vi "nnfft.vi"() -> ()   [LabVIEW 2014]
uses:
  <vilib>/imath/engines/lvmath/Functions/Error Handling/error.ctl
  <vilib>/Analysis/baseanly.llb/Real A x B.vi
  <vilib>/DAQmx/create/channels.llb/DAQmx Create Channel (AI-Voltage-Basic).vi
  <vilib>/DAQmx/create/channels.llb/DAQmx Create Channel (DO-Digital Output).vi
  <vilib>/imath/engines/lvmath2/RunTimeEngine/Managers/WorkSpace/UID Generator.vi
  <vilib>/imath/engines/lvmath2/RunTimeEngine/NonStaticBuiltInFunctions/Manual/NIMS_NS_load.vi
  <vilib>/imath/engines/lvmath/Plug In/Control Design/NonStaticBuiltInFunctions/NIMS_NS_length.vi
  <vilib>/imath/engines/lvmath/Plug In/_Char/NIMS_CH_String to Character Array.vi
  <vilib>/imath/engines/lvmath2/RunTimeEngine/RunTimeType/NIMS_RunTimeType_From StrictType (excl LVString).vi
  <instcachedir>/0/NIMS_RunTimeType_From StrictType (excl LVString)_15A5391EEA9C4AACB9955AC755B83D29.lvgen/NIMS_RunTimeType_From StrictType (excl LVString)_15A5391EEA9C4AACB9955AC755B83D29_001.vi
  <vilib>/imath/engines/lvmath2/RunTimeEngine/Managers/SymbolTable/Write Variable.vi
  <vilib>/imath/engines/lvmath2/RunTimeEngine/RunTimeSymbolToken/NIMS_RunTimeSymbolToken_ReadVariable-1out.vi
  <vilib>/imath/engines/lvmath/Plug In/Control Design/RunTimeSymbolToken/NIMS_CD_RunTimeSymbolToken_ResolveSymbol.vi
  <instcachedir>/0/NIMS_CD_RunTimeSymbolToken_ResolveSymbol_41E3A8865B50468190B6702AA519A4CE.lvgen/NIMS_CD_RunTimeSymbolToken_ResolveSymbol_41E3A8865B50468190B6702AA519A4CE_000.vi
  <instcachedir>/0/NIMS_CD_RunTimeSymbolToken_ResolveSymbol_41E3A8865B50468190B6702AA519A4CE.lvgen/NIMS_CD_RunTimeSymbolToken_ResolveSymbol_41E3A8865B50468190B6702AA519A4CE_001.vi
  <vilib>/imath/engines/lvmath/Plug In/Control Design/RunTimeSymbolToken/NIMS_CD_RunTimeSymbolToken_ResolveUDForVariable-1out.vi
  <vilib>/imath/engines/lvmath/Plug In/Control Design/ArithmeticOperatorToken/NIMS_CD_NS_ArithmeticOperator_minus.vi
  <vilib>/imath/engines/lvmath/Plug In/Control Design/ArithmeticOperatorToken/NIMS_CD_NS_ArithmeticOperator_cctranspose.vi
  <vilib>/imath/engines/lvmath2/RunTimeEngine/CommandStatement/NIMS_CommandStatement_MaskErr.vi
  <vilib>/imath/engines/lvmath2/RunTimeEngine/Managers/SymbolTable/Read Variable.vi
  <vilib>/imath/engines/lvmath2/RunTimeEngine/RunTimeType/NIMS_RunTimeType_Get Case Value.vi
  <vilib>/imathl/engines/lvmath/Functions/Error Handling/Create Error.vi
  <vilib>/imath/engines/lvmath2/RunTimeEngine/RunTimeType/NIMS_RunTimeType_To Numeric.vi
  <instcachedir>/0/NIMS_RunTimeType_To Numeric_CEDD3DBADEB64FB59CD8C53099B6B149.lvgen/NIMS_RunTimeType_To Numeric_CEDD3DBADEB64FB59CD8C53099B6B149_000.vi
  <vilib>/imath/engines/lvmath2/RunTimeEngine/NodeEndStatement/NIMS_NodeEndStatement_Get Scalar.vi
  <instcachedir>/0/NIMS_NodeEndStatement_Get Scalar_62223508BC7F4CFFA0F66459A43A6646.lvgen/NIMS_NodeEndStatement_Get Scalar_62223508BC7F4CFFA0F66459A43A6646_000.vi
  <vilib>/imath/engines/lvmath/Plug In/_Char/RunTimeType/NIMS_CH_RunTimeType_To Character 2D.vi
  <instcachedir>/0/NIMS_NodeEndStatement_Get Scalar_62223508BC7F4CFFA0F66459A43A6646.lvgen/NIMS_NodeEndStatement_Get Scalar_62223508BC7F4CFFA0F66459A43A6646_001.vi
  <vilib>/Analysis/Matrix/Numeric/Conversions/Array To Matrix - RA2.vi
  <vilib>/imath/engines/lvmath/Plug In/_Char/NIMS_CH_Character 2D to U8 2D.vi
  <vilib>/imath/engines/lvmath/Functions/Error Handling/MergeErrorsWrapper.vi
  <vilib>/imath/engines/lvmath2/RunTimeEngine/NodeEndStatement/MC_NodeEndStatement_Dispose.vi
  <vilib>/imath/engines/lvmath2/RunTimeEngine/NodeEndStatement/NIMS_NodeEndStatement_Output.vi
  <instcachedir>/0/NIMS_NodeEndStatement_Output_53EC0D466D134D7ABD903AC30B43404B.lvgen/NIMS_NodeEndStatement_Output_53EC0D466D134D7ABD903AC30B43404B_013.vi
  <instcachedir>/0/NIMS_NodeEndStatement_Output_53EC0D466D134D7ABD903AC30B43404B.lvgen/NIMS_NodeEndStatement_Output_53EC0D466D134D7ABD903AC30B43404B_011.vi
  <instcachedir>/0/NIMS_NodeEndStatement_Output_53EC0D466D134D7ABD903AC30B43404B.lvgen/NIMS_NodeEndStatement_Output_53EC0D466D134D7ABD903AC30B43404B_001.vi
  <instcachedir>/0/NIMS_NodeEndStatement_Output_53EC0D466D134D7ABD903AC30B43404B.lvgen/NIMS_NodeEndStatement_Output_53EC0D466D134D7ABD903AC30B43404B_012.vi
  <vilib>/imath/engines/lvmath2/RunTimeEngine/ErrorHandling/NIMS_Finalize Error.vi
  <vilib>/DAQmx/configure/timing.llb/DAQmx Timing (Sample Clock).vi
  <vilib>/DAQmx/read.llb/DAQmx Read (Analog 1D Wfm NChan NSamp).vi
  <vilib>/express/express analysis/Spectral/Block/exnSpectralBlock spectral measurements PSD poly.vi
  <vilib>/express/express analysis/Spectral/Block/exnSpectralBlock spectral measurements PSD WFM.vi
  <vilib>/Analysis/Matrix/Numeric/Conversions/Array To Matrix - RA.vi
  <vilib>/Analysis/Matrix/Numeric/Add/Add - RM,RM.vi
  <vilib>/DAQmx/write.llb/DAQmx Write (Digital 2D Bool NChan 1Samp NLine).vi
  <vilib>/express/express analysis/Spectral/XNode/ExpressSpectralMeasurementsBlockNode.xnode
  <vilib>/Analysis/Matrix/NI_Matrix.lvlib
  <vilib>/Analysis/NI_AALBase.lvlib
  <vilib>/imath/engines/lvmath2/RunTimeEngine/Managers/SymbolTable/NIMS_WorkSpace.lvlib
panel:
  out "detected signal":i16[][](graph)
  out "Max power":dbl
  out "Waveform Chart":waveform(dbl)[](graph)
  out "canonical signal":i16(graph)
  in  "Path":path=path "Z:/v/birds/align/net_detector_0.28_0.775.mat"
  in  "stop":bool
  out "FFT_TIME_SHIFT":dbl=0.005
  out "FFT_SIZE":i32=256
  out "samplerate":dbl=24414.0625
  out "window":dbl[][](graph)=[[-72.97635032393673, -73.52535220045053, -65.72887335245875, -68.76871345390529, -72.8382109706844, -72.4284168123761, -76.29548482618758, -74.74287956205296, -81.97895834534424, -76.96305090475649, -75.98014073911352, -80.03992621585844, -83.84107312947093, -89.59209404799233, -79.87440020414152, -81.36512283954667, -88.18744053916166, -81.6924166622812, -77.53707705274705, -86.56451602394448, -79.73285708058553, -74.22115387848037, -71.41210134154478, -74.47517384018045, -74.77033095311324, -80.80005153541933, -80.79191388333305, -77.97946550843649, -75.05698688298563, -77.91422524584947, -81.26748634507513, -78.23409719434568, -71.56701464425281, -69.17263385066326, -77.53908052412173, -75.51920407149245, -72.81493380643417, -75.82836580399663, -79.16788759874976, -85.18140498406765, -73.69950641565677, -77.89257807943649, -89.09322579355587, -86.98629885093659, -82.38468041348978, -80.6411265118298, -82.76696738280094, -88.62107664481837, -80.16920149619398, -87.78502444899082, -76.5547272830016, -79.26058810386263, -83.94947298172212], [-66.67637324595356, -64.45280082019433, -72.37911061109125, -80.94357987532189, -72.53604430129853, -77.45470711834774, -89.59806575492826, -76.48927163271915, -73.61448223145683, -73.49144401291508, -71.27370666896533, -71.20261780246133, -74.92587625827385, -74.29334726263828, -76.65530048928724, -82.00140588849537, -79.57538322888249, -77.80520492576613, -81.78737082190267, -81.793811852895, -76.25688370577186, -78.13061054962415, -79.77815579754174, -74.3873327071945, -75.70646544653732, -90.72121289782154, -78.03321007215462, -81.03438405652348, -79.87658452660123, -76.00205540897467, -89.87308398872139, -81.86767670866956, -76.2852996579092, -70.93465158513496, -71.34523644690213, -79.93221348833194, -92.79662932893322, -79.70914845480407, -80.2829643889263, -84.90892181441768, -76.68651665541584, -84.51267326878296, -82.8204756496925, -76.73565845150263, -73.04092896348672, -74.3315440085461, -78.03729006688118, -81.70866916339699, -92.11943263220843, -79.10810077302251, -80.08002292830199, -86.99321689797517, -85.04323742707173], [-60.36185307894806, -67.68102358288463, -73.44778253010914, -83.24181048562586, -73.96144044519264, -84.69635305857125, -81.14261573322445, -79.25621064770326, -76.529695092035, -75.04627154406595, -73.90530564973237, -75.82555328376658, -72.10380949692679, -75.32839456413583, -76.50304991511011, -75.65339129055367, -77.00187973819256, -76.57898166561162, -82.8025996290185, -73.19174517705048, -69.09785163927901, -67.53276211170689, -72.94360264826646, -79.97186045768333, -88.56886550153519, -88.83521591582405, -76.65307428710892, -73.00745577396138, -74.258180742689, -71.06328438122829, -72.78097301088393, -76.66465643284776, -81.62018899033966, -75.65821895156606, -82.17348753133518, -80.91069867191484, -70.46021775773852, -68.83368607770463, -69.03429126209139, -72.72415945910303, -73.80156036987256, -69.28349217732242, -68.01356058946793, -73.4812440368461, -75.17978018102508, -77.01602519651868, -73.18724221539284, -73.00676255493443, -71.9944333961078, -72.09084959215544, -78.65722374826107, -76.66612517006482, -74.38697175839361], [-86.00798842509802, -75.66491243286761, -69.45998734378524, -75.90898538704424, -71.26588425831507, -68.18490140120666, -76.40500842112715, -90.04695090636658, -75.34084116331435, -73.50738067142525, -78.60366511108383, -81.21647416858836, -78.9684969474276, -82.40208977563746, -73.24305990075133, -71.12237211198403, -82.91234590794866, -80.93715499149765, -78.06474769268046, -75.91020347678767, -81.60811248967987, -82.86113678420863, -76.87398598776707, -74.38664233198445, -71.82140107556668, -74.67033624127943, -78.17390364475995, -72.60207540814541, -71.04336646832618, -67.87557323613137, -67.16318617639155, -69.4250953016462, -71.39893400102616, -68.4807322912351, -82.25308112419869, -68.3200120825788, -69.81250624283365, -71.84163203711881, -66.75402172042715, -86.50070599392079, -68.88587550717388, -64.27484144399455, -63.21158787522782, -66.63527192363303, -67.84532057406827, -66.45376461718031, -67.62579522979001, -70.50214513926198, -67.25446907463098, -65.19333416310778, -69.41880953289862, -71.51704770295385, -69.35219267630163], [-84.02423956482974, -80.30370937609739, -72.07006291884605, -78.91836472420934, -68.25364204650245, -76.68501322644221, -75.18375824555125, -71.83467956160965, -70.95375248124259, -74.08077326369566, -67.38027814308849, -72.93566891736185, -67.65115715678446, -64.85035252961103, -64.82034005578986, -70.26034479840374, -70.45877563236849, -76.54420720294256, -81.78534267236304, -78.15256514501289, -82.91835245277196, -72.46741612058328, -73.68274550784452, -78.34739661909776, -78.9666065362011, -77.78534451234053, -74.37093982228039, -74.12317719447532, -78.16971177499396, -74.52074730296583, -76.54045500868807, -75.84578212694746, -74.67082902652055, -77.18938861537275, -69.907454938437, -75.34017205802814, -79.50572953621057, -72.34299872242158, -78.18111149918124, -75.54782414585868, -80.561212592933, -75.11175049302021, -75.69417919582135, -78.60245860449001, -95.87767775375552, -87.11569980194378, -85.92469188794526, -77.60906632245548, -71.79465409556695, -77.42305609850067, -83.12532465877507, -77.05370659978007, -79.71270482455323], [-81.65381289229904, -83.21306508163494, -79.67200080348587, -70.22488500380918, -67.822116429376, -66.63216387482694, -69.55869616362561, -81.4902489378859, -78.79527713122093, -67.33672711847055, -60.3507452058667, -58.73683599716651, -60.551256165403004, -64.32429540525435, -64.72915177181335, -66.22450762492544, -91.58683040813399, -84.38309032351134, -73.15703222555902, -67.56828517210809, -73.57402369414261, -74.61227498203642, -77.96234972672107, -71.20169596754377, -67.59425187404017, -71.05072968837761, -76.59202882173123, -80.82688050565231, -73.80977565569785, -74.11008150826325, -71.41495591144026, -77.7753259840453, -76.2037224219869, -79.29218960734961, -91.32887569169418, -85.7301249007533, -80.85079471385804, -74.18909859098636, -72.26476740645808, -73.32812816132918, -75.76304038496815, -77.50309269541718, -73.05090728588225, -71.86574972197677, -70.43058663023983, -70.27591438296898, -74.08700994335328, -73.95177555941575, -91.88200670928885, -81.81331742651899, -78.5318263177664, -71.72863325861373, -74.46402142105174], [-68.9073260193967, -67.48746628924823, -77.17977545292486, -73.64769729099787, -72.22314785727713, -70.87731592806281, -70.716894114705, -81.05789728768389, -71.43183739761903, -73.18594956271083, -69.20692855319716, -68.67815172293385, -53.670962574687195, -50.933292802391094, -61.63077047269332, -71.38477936140977, -99.14569301468815, -72.06562278900773, -74.1511754276874, -76.89887661322872, -72.58638083106267, -75.05922049222346, -77.77343214730914, -75.92379207288955, -71.20325396519463, -76.43168692677789, -82.39119805432924, -71.51193816622407, -73.1364143798586, -78.71213040493862, -94.96695151435625, -74.49648076734441, -69.43231860114312, -70.3883036388338, -76.6904252867458, -85.10664073795765, -83.20367116345437, -79.50305757838471, -74.03353087441471, -78.99092469951292, -91.58509571109497, -91.89444165362694, -79.83050377520397, -79.27431251753544, -84.8477925073274, -72.43027174269308, -65.52053141156405, -66.12640598342038, -76.108195822798, -89.27574855580932, -70.90463844447619, -66.46347719708304, -72.98967833873088], [-73.0439648592936, -70.44453567604373, -79.75314488295, -80.07642120248778, -78.37070295298031, -73.1201693139319, -78.53710949103558, -79.79936428129609, -79.86525021136373, -72.22971430283177, -67.84318418359742, -72.87558430802864, -53.003002816738515, -47.84968331998619, -50.98562535099076, -58.11218860294475, -61.60082326832688, -68.69125001358182, -70.44497259313596, -69.84352221154673, -72.07552086745858, -73.19525392036374, -85.84209460576159, -78.78668117995774, -108.96094371547589, -76.45977938927919, -75.02269494673682, -81.13939454241775, -76.23809744857965, -79.98125590046457, -85.47323069676317, -82.94387240494945, -77.0798993807903, -87.45325755760888, -74.60902178190632, -71.49002838584563, -72.65326888909527, -74.30285347007833, -71.51996549981243, -70.58127271813062, -67.50879993296408, -66.96776504010182, -67.5977737300707, -63.43592929677993, -65.07886006448592, -68.14664606850042, -65.25796945257115, -63.375993543512465, -69.69409051293428, -66.76473458025286, -67.28346558898642, -70.59116729035524, -67.66948910837607], [-68.77569667006642, -69.18302500016709, -71.01858086817602, -72.38028122261937, -69.84097809370121, -70.94893664271633, -76.08982385135212, -78.69559608023533, -75.44131958210247, -70.6072977643919, -68.94517408706297, -69.39438458347952, -63.31192689032822, -62.17555246766285, -67.17754626637941, -75.62442591074503, -78.75800065905979, -75.17375793297293, -73.35352004961631, -76.14826387288446, -76.94316620614036, -82.59526691265685, -71.38733095904792, -72.56519374181563, -83.3950501348429, -90.47654618015734, -84.51605264553925, -75.11223707596085, -75.67115447672266, -79.48878198359742, -72.8312370379487, -73.12224612826401, -73.48400779569472, -72.78689045619967, -76.92547768121204, -78.40592890718482, -73.2310717836559, -66.03581732569029, -72.47607194397511, -63.68851741665692, -64.64949331188906, -58.02441919784529, -59.84253402809921, -55.317855401116205, -55.64943410315087, -55.07048062012055, -53.75573935219861, -59.01222904078905, -56.55051323885307, -55.924357615058895, -55.62810503061498, -54.23211672544804, -55.50519500194375], [-74.75832710617124, -75.4308719211877, -74.46594285292588, -73.08174465947688, -75.65741389741267, -76.85655422277733, -76.17724583134641, -78.7866469753405, -79.98861317568219, -81.89112371724251, -82.63604725769618, -83.140254780378, -81.67601959545613, -89.00653003380093, -88.73873918927613, -76.51543291625471, -75.79644478079794, -80.51350580935683, -78.29033538027453, -77.6006603336961, -82.29627474182139, -78.33191904398069, -75.62832998601185, -86.33820054880604, -78.0946880670678, -74.84100282711086, -75.24721439405523, -78.59378634737459, -82.46985087316023, -79.76367779929939, -83.59485868627448, -74.82964327789745, -83.47070996793212, -80.84481800459685, -88.96399452691867, -76.9164788840067, -70.71773824416289, -68.11387991161286, -84.5841447765394, -66.7959107046369, -68.75178657989372, -64.77026879341615, -67.70334881108903, -53.99229230247266, -54.15690890913606, -51.07210226513892, -47.4469848829612, -48.016313760511224, -46.89883581264472, -47.32639944655021, -47.087219879398575, -49.520586995280375, -51.40004089705311], [-84.80810487129318, -80.63211281718762, -78.56043117891872, -76.27943201998615, -77.15760293197748, -81.64091579144285, -83.57045080108676, -78.63130196693999, -81.47341405888328, -78.60904777055399, -78.00888189113262, -85.12607813424106, -83.64938163698022, -80.79078185456909, -81.96965893927523, -77.43741043097695, -78.52875304218192, -79.13790302072155, -79.8115060848578, -89.09700475707078, -79.84774992179518, -81.4208933359674, -79.45746012306984, -82.24946297830411, -87.56044829973484, -90.28729530511617, -76.44434861584307, -78.78897610507829, -93.34714140321714, -79.6437809904397, -77.08007637946908, -82.61823969652897, -96.96492301906731, -86.91840996208597, -78.2484679644696, -84.06167675912474, -80.58283631847846, -82.60282000113612, -80.08784422911889, -80.3818141223883, -71.63670327697784, -71.70751698739937, -76.76453620599743, -71.61768539867478, -69.32504730623252, -68.28032804698583, -65.759956184971, -65.61488756706426, -65.70881887875339, -67.262085308336, -71.32336101600086, -73.79617107128622, -74.47767495897709], [-74.24876447880565, -79.51183675628256, -89.46410450431294, -82.92587289022006, -77.7457556235718, -79.30413919682815, -80.50830335354752, -81.3585175894736, -71.63315075617669, -71.50011424611691, -78.47849160378934, -80.30674914126804, -73.11186901485297, -76.026499122226, -78.67243959562191, -81.28052088875201, -77.39332987892728, -79.17775124486431, -74.63358089302206, -74.2219431039591, -75.72536721687463, -78.63557830761712, -78.03300701227882, -78.73460743340698, -80.50182310318193, -74.34525414950886, -78.93836541260941, -97.94071592484138, -91.61898811661828, -78.45177452289117, -79.02722537868969, -87.81919073287318, -97.64889457820716, -86.08948913346865, -94.83472004300674, -80.29958208150036, -79.94308117838753, -87.26408456051925, -87.86724547094477, -77.22219882470283, -79.10106862704167, -81.9160924832359, -75.92381304866126, -79.29802559293336, -78.63678572865807, -80.2339821401618, -80.74035656476087, -75.34996964522848, -74.87202873304834, -76.5943391889857, -73.41497745912935, -75.30585362948747, -82.47751215796093], [-74.39306178800754, -73.02600059267387, -73.07393952038746, -74.9812550588737, -76.80613423181211, -79.21537174139556, -82.24804461952566, -79.88497680349332, -77.73780357707737, -76.38987395680789, -81.1372862629103, -84.67801257122353, -75.29730335181587, -84.00023147835932, -73.3237703431372, -74.21062661277206, -80.51423062939938, -73.23425723998423, -72.49958681733966, -80.41967028089522, -88.8780775783741, -79.02412566482069, -90.7377774207196, -73.42552841442792, -74.68738171044559, -73.67460705564318, -76.06590490239931, -84.7613317932862, -79.70125370326343, -79.49333540467144, -89.63642567674898, -83.03621171058427, -83.33948920260524, -82.46001987798482, -81.95215264151247, -85.35054456568888, -86.49328712600567, -81.97249680506789, -87.5387622178776, -85.66227087431446, -84.18576775722295, -80.40800661446254, -75.53107385453657, -82.15686513878657, -88.67483064056772, -87.66221780558206, -86.84772744676606, -79.53573628729012, -82.7762696782156, -80.7915757346325, -80.70452295791704, -85.6983850384739, -81.72315222245822], [-81.93627780778903, -76.28366916681793, -80.29872988619105, -87.05275862910486, -84.63141287821459, -77.18015134120228, -72.98884655283919, -75.52679661054356, -80.1056525653624, -74.6697942063844, -80.48729503314061, -75.50337131233141, -78.31665631669648, -82.43718806714023, -73.95226171890097, -72.9292996254482, -71.71861568455955, -80.7946502972628, -78.65549947452148, -76.96606097973789, -76.06401494770057, -75.97723913018525, -99.24458365039294, -75.64074011120537, -78.62239631692377, -86.48850642086873, -89.87032184925617, -82.76174629794922, -80.10136504583882, -79.9961860071702, -81.50677446791065, -84.25440065532206, -92.56018408560594, -83.18151695684361, -80.59299994282482, -83.02918337502582, -78.40907071643018, -77.83883198956002, -89.31961651857968, -76.63471365127987, -75.67292636105336, -81.12402945042773, -90.28605099784328, -79.706246286267, -84.4032682475605, -81.20491587848613, -83.58829972237129, -92.4308955170453, -114.2328518473521, -78.71042595894347, -73.75405245226335, -74.69214248881669, -80.75531088405972]]
  out "Full spectrogram":dbl[][](graph)=[[-60.61401215305423, -57.03689977091529, -62.342730493983005, -72.51114353592169, -76.22824519389013, -78.52855635448381, -79.58628749191288, -67.73644127838553, -68.84105664914598, -74.67612003437475, -75.63706315714897, -76.74817498515577, -78.32477078138152, -73.09465183010549, -84.9742009024476, -82.47248060505194, -73.7376673139534, -68.19154425689516, -69.20475014657619, -88.95954172279392, -72.41169373066344, -81.93627780778903, -76.28366916681793, -80.29872988619105, -87.05275862910486, -84.63141287821459, -77.18015134120228, -72.98884655283919, -75.52679661054356, -80.1056525653624, -74.6697942063844, -80.48729503314061, -75.50337131233141, -78.31665631669648, -82.43718806714023, -73.95226171890097, -72.9292996254482, -71.71861568455955, -80.7946502972628, -78.65549947452148, -76.96606097973789, -76.06401494770057, -75.97723913018525, -99.24458365039294, -75.64074011120537, -78.62239631692377, -86.48850642086873, -89.87032184925617, -82.76174629794922, -80.10136504583882, -79.9961860071702, -81.50677446791065, -84.25440065532206, -92.56018408560594, -83.18151695684361, -80.59299994282482, -83.02918337502582, -78.40907071643018, -77.83883198956002, -89.31961651857968, -76.63471365127987, -75.67292636105336, -81.12402945042773, -90.28605099784328, -79.706246286267, -84.4032682475605, -81.20491587848613, -83.58829972237129, -92.4308955170453, -114.2328518473521, -78.71042595894347, -73.75405245226335, -74.69214248881669, -80.75531088405972, -82.82888754576534, -82.01868690982059, -81.78786972713498, -82.23423354778731, -78.28473979595428, -80.87670751550114, -83.51180745110783, -82.69187002570317, -88.82008519429516, -75.98520288801285, -77.99668488932495, -87.62318296403504, -99.6141881068977, -81.81521098057642, -84.17434860926062, -76.06411102913623, -74.1198176945056, -81.12819699144072, -80.91815093081088, -78.14119584663972, -85.49724935291657, -91.38248083630508, -84.18310225258782, -84.77684376955226, -85.16944043858439, -79.9875938684393, -79.27633537810411, -81.02037581981868, -81.35173013966018, -96.42412550048378, -90.54677478925467, -87.40674735535208, -88.1750427749852, -81.74631327698087, -82.23000371533317, -81.3297319022112, -76.40113644324768, -87.80400336917077, -78.37126070791032, -83.49976513431899, -80.51126278317908, -78.30520883073534, -76.75167662319735, -75.54421920890346, -79.45387512183294, -79.23147015013464, -82.63339787200022, -84.67740230235428, -67.26543692771294, -65.23077893430924, -76.87705017438371, -86.75690272003072, -85.56129846796406, -79.28978800654977]]
  out "in-loop read error":errorcluster
  out "daq create error":errorcluster
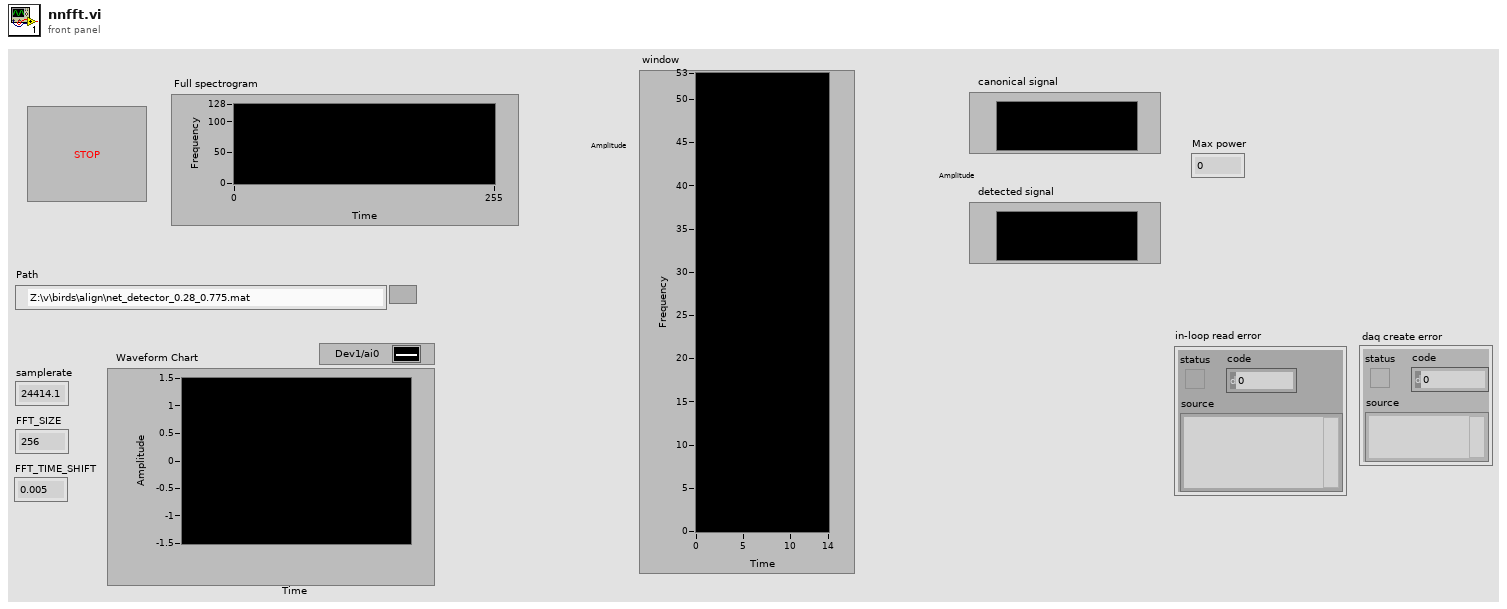
[diagram p1: front panel]
types:
  T1 = typedef "NI_Matrix.lvlib/RealMatrix.ctl" = dbl[][]
  T2 = cluster{"averaging mode":u16, "weighting mode":u16, "number of averages":u32}
  T3 = cluster{"dB On (F)":bool, "unwrap phase (F)":bool, "convert to degree (F)":bool}
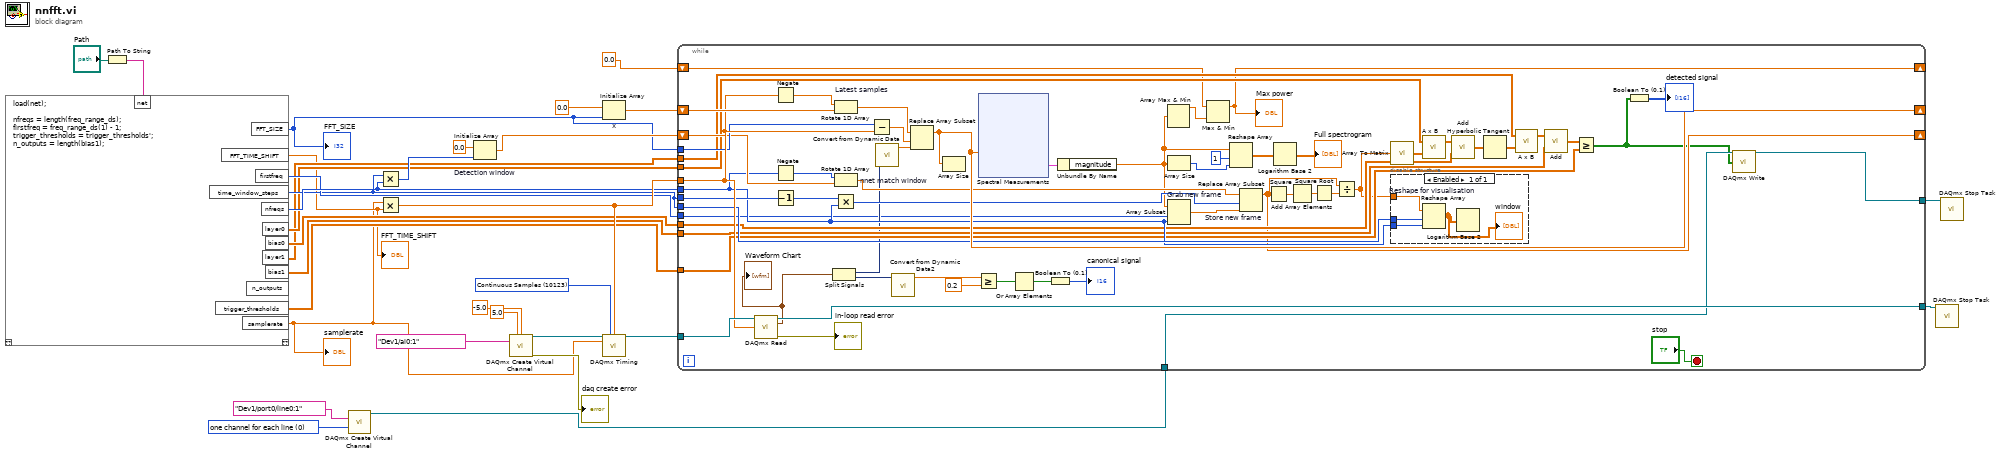
[diagram p0: block diagram]
diagram:
  w5 = 0 items=["one channel for each line", "one channel for all lines"] ("line grouping")
  w29 = 10123 items=["Finite Samples"=10178, "Continuous Samples"=10123, "Hardware Timed Single Point"=12522] ("sample mode")
  n1 = Path To String(path="Path") -> (string=w9:string)
  n2 = mathscript code="load(net);\n\nnfreqs = length(freq_range_ds);\nfirstfreq = freq_range_ds(1) - 1;\ntrigger_thresholds = trigger_thresholds';\nn_outputs = length(bias1);"("net"=w9) -> ("FFT_TIME_SHIFT"=w12:dbl, "firstfreq"=w19:i32, "time_window_steps"=w18:i32, "nfreqs"=w20:i32, "layer0"=w17:T1, "bias0"=w16:T1, "layer1"=w15:T1, "bias1"=w14:T1, "trigger_thresholds"=w13:T1, "samplerate"=w10:dbl, "FFT_SIZE"=w11:i32)  [unwired: 1 in, 2 out]
  "samplerate" <- w10
  "FFT_SIZE" <- w11
  "FFT_TIME_SHIFT" <- w12
  n3 = call-poly <vilib>:"DAQmx Create Virtual Channel.vi"("lines"=tag "Dev1/port0/line0:1", "line grouping"=w5) -> ("task out"=w7:refnum<k21>)  [unwired: 12 in, 1 out]
  n4 = Multiply(x=w18, y=w20) -> (x*y=w22:i32)
  n5 = Multiply(x=w10, y=w12) -> (x*y=w27:dbl)
  n6 = Initialize Array "Detection window"(0.0 ("element"), w22) -> (w21:dbl[])
  n7 = call-poly <vilib>:"DAQmx Create Virtual Channel.vi"("maximum value"=5.0, "minimum value"=-5.0, "physical channels"=tag "Dev1/ai0:1") -> ("task out"=w32:refnum<k21>, "error out"=→"daq create error":errorcluster)  [unwired: 11 in]
  n8 = Initialize Array "x"(0.0 ("element"), w11) -> (w24:dbl[])
  n9 = call-poly <vilib>:"DAQmx Timing.vi"("task/channels in"=w32, "sample mode"=w29, "samples per channel"=w27, "rate"=w10) -> ("task out"=w25:refnum<k21>)  [unwired: 10 in, 1 out]
  n10 = while {
    tunnel: w11 -> [w82]
    tunnel: w27 -> [w84]
    tunnel: w25 -> [w89]
    tunnel: [w90] -> w26
    shift-right: [w86] -> _
    shift-left: w24 -> [w88]
    shift-right: [w37] -> _
    shift-left: w21 -> [w78]
    tunnel: w20 -> [w70]
    tunnel: w18 -> [w74]
    tunnel: w19 -> [w33]
    tunnel: w18 -> [w71]
    tunnel: w17 -> [w68]
    tunnel: w16 -> [w66]
    tunnel: w15 -> [w60]
    tunnel: w14 -> [w63]
    tunnel: w13 -> [w58]
    tunnel: w7 -> [w57]
    tunnel: [w56] -> w6
    shift-right: [w45] -> _
    shift-left: 0.0 -> [w46]
    stop <- "stop" stop-if-true
    n11 = call-poly <vilib>:"DAQmx Read.vi"("task/channels in"=w89, "number of samples per channel"=w84) -> ("task out"=w90:refnum<k21>, "data"=w34:waveform(dbl)[], "error out"=→"in-loop read error":errorcluster)  [unwired: 11 in]
    "Waveform Chart" <- w34
    n12 = Negate(x=w84) -> (-x=w83:dbl)
    n13 = Negate(x=w70) -> (-x=w77:i32)
    n14 = Decrement(x=w74) -> (x-1=w73:i32)
    n15 = Split Signals(w34) -> (w43:dynamicdata, w42:dynamicdata)  [unwired: 2 in]
    n16 = Rotate 1D Array "Latest samples"(1:w88, 2:w83) -> (0:w87:dbl[])
    n17 = Rotate 1D Array "nnet match window"(1:w78, 2:w77) -> (0:w76:dbl[])
    n18 = Multiply(x=w73, y=w70) -> (x*y=w72:i32)
    n19 = Subtract(x=w82, y=w84) -> (x-y=w85:dbl)
    n20 = call "Convert from Dynamic Data"("Dynamic Data Type"=w43) -> ("Array"=w55:dbl[])  [unwired: 3 in]
    n21 = call "Convert from Dynamic Data2"("Dynamic Data Type"=w42) -> ("Array"=w54:dbl[])  [unwired: 3 in]
    n22 = Replace Array Subset(array=w87, new element=w55, index=w85) -> (w86:dbl[])
    n23 = Array Size(array=w86) -> ()  [unwired: 1 out]
    n24 = Greater Or Equal?(x=w54, y=0.2) -> (x >= y?=w53:bool[])
    n25 = xnode "Spectral Measurements"("Signals"=w86) -> ("PSD"=w80:cluster{"f0":dbl, "df":dbl, "magnitude":dbl[]})  [unwired: 1 in, 1 out]
    n26 = Or Array Elements(Boolean array=w53) -> (logical OR=w52:bool)
    n27 = Boolean To (0,1)(Boolean=w52) -> (0, 1=→"canonical signal":i16)
    n28 = Unbundle By Name(w80) -> ("magnitude"=w48:dbl[])
    n29 = Array Max & Min(array=w48) -> (max value=w47:dbl)  [unwired: 3 out]
    n30 = Array Size(array=w48) -> (size(s)=w79:i32)
    n31 = Array Subset "Grab new frame"(array=w48, index=w33, length=w70) -> (w75:dbl[])
    n32 = Max & Min(x=w46, y=w47) -> (max(x,y)=w45:dbl)  [unwired: 1 out]
    "Max power" <- w45
    n33 = Reshape Array(w48, 1 ("dimension size"), w79) -> (w49:dbl[][])
    n34 = Replace Array Subset "Store new frame"(array=w76, new element=w75, index=w72) -> (w37:dbl[])
    n35 = Square(x=w37) -> (x^2=w41:dbl[])
    n36 = Logarithm Base 2(1:w49) -> (0:→"Full spectrogram":dbl[][])
    n37 = Add Array Elements(numeric array=w41) -> (sum=w40:dbl)
    n38 = Square Root(x=w40) -> (sqrt(x)=w39:dbl)
    n39 = Divide(x=w37, y=w39) -> (x/y=w38:dbl[])
    n40 = call-poly <vilib>:"Array To Matrix.vi"("Real 1D Array"=w38) -> ("Real Matrix (Column Vector)"=w69:T1)
    n41 = disable-structure shown="Enabled" {
      disable-tunnel: w38 -> [w95]
      disable-tunnel: w71 -> [w94]
      disable-tunnel: w70 -> [w93]
      frame Enabled {
        n42 = Reshape Array "Reshape for visualisation"(w95, w94, w93) -> (w92:dbl[][])
        "window" <- w92
        n43 = Logarithm Base 2(1:w92) -> ()  [unwired: 1 out]
      }
    }
    n44 = call-poly <vilib>:"A x B.vi"("B"=w69, "A"=w68) -> ("A x B"=w67:T1)  [unwired: 1 out]
    n45 = call-poly <vilib>:"Add.vi"("Real Matrix B"=w66, "Real Matrix A"=w67) -> ("A + B"=w65:T1)
    n46 = Hyperbolic Tangent(1:w65) -> (0:w61:T1)
    n47 = call-poly <vilib>:"A x B.vi"("B"=w61, "A"=w60) -> ("A x B"=w64:T1)  [unwired: 1 out]
    n48 = call-poly <vilib>:"Add.vi"("Real Matrix B"=w63, "Real Matrix A"=w64) -> ("A + B"=w59:T1)
    n49 = Greater Or Equal?(x=w59, y=w58) -> (x >= y?=w35:bool[][])
    n50 = Boolean To (0,1)(Boolean=w35) -> (0, 1=→"detected signal":i16[][])
    n51 = call-poly <vilib>:"DAQmx Write.vi"("task/channels in"=w57, "data"=w35) -> ("task out"=w56:refnum<k21>)  [unwired: 11 in, 2 out]
  }
  n52 = call <vilib>:"DAQmx Stop Task.vi"("task/channels in"=w26) -> ()  [unwired: 13 in, 2 out]
  n53 = call <vilib>:"DAQmx Stop Task.vi"("task/channels in"=w6) -> ()  [unwired: 13 in, 2 out]
